vi "SetGTI.vi"(1 "gti_mode":u8, 2 "drv":u32) -> ()   [LabVIEW 2015]
uses:
  ESLSCDLL.dll
panel:
  # "Chooses trigger input for general trigger input (GTI)\t\n- 0: I\n\t- 1: S1\n\t- 2: S2\n\t- 3: GND"
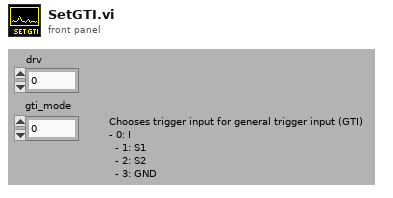
[diagram p1: front panel]
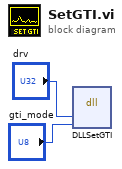
[diagram p0: block diagram]
diagram:
  n1 = dll-call lib="C:/ENTW/PCIE/lv64/board.vis/ESLSCDLL.dll" fn="DLLSetGTI" ("lwlscdll.dll:DLLRsTOREG")("drv"="drv", "gti_mode"="gti_mode") -> ()  [unwired: 6 in, 2 out]
